vi "GetParam.vi"(8 "error in (no error)":errorcluster caption="entrée d'erreur (pas d'erreur)", 11 "GroupKFold.lvclass":refnum<class "GroupKFold.lvclass">) -> (0 "error out":errorcluster caption="sortie d'erreur", 2 "GroupKFold":cluster{"n_splits":i32}={"n_splits"=5}, 3 "GroupKFold.lvclass":refnum<class "GroupKFold.lvclass">)   [LabVIEW 2020, in "GroupKFold.lvclass"]
doc: "Get Parameters"
uses:
  GroupKFold.lvclass
  GroupKFold.lvclass/GroupKFold.ctl
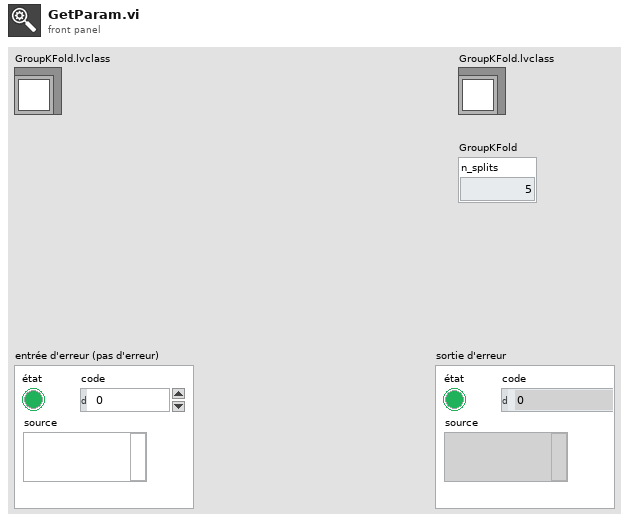
[diagram p1: front panel]
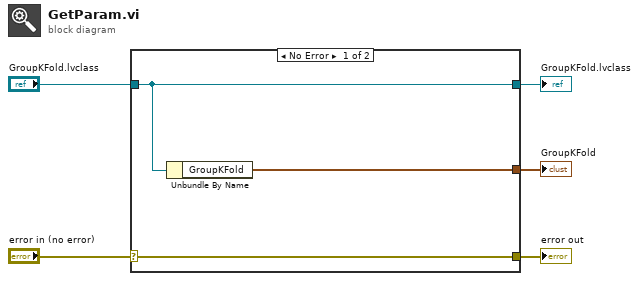
[diagram p0: block diagram]
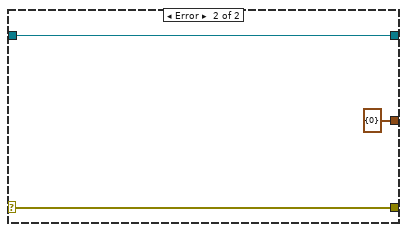
[diagram p2: hidden frame]
diagram:
  n1 = case shown="No Error" "error in (no error)" {
    selector: "error in (no error)" -> [w8 w10]
    tunnel: [w8 w10] -> w4
    tunnel: [w7 w11] -> w2
    tunnel: "GroupKFold.lvclass" -> [w7 w11]
    tunnel: [w6 cluster{"n_splits":i32} {"n_splits"=0} ("GroupKFold")] -> w1
    frame No Error {
      n2 = Unbundle By Name(w7) -> ("GroupKFold"=w6:cluster{"n_splits":i32})
    }
    frame Error {
    }
  }
  "error out" <- w4
  "GroupKFold.lvclass" <- w2
  "GroupKFold" <- w1
